vi "GET_LayersLocked_ActiveLayer.vi"(8 "error in (no error)":errorcluster, 11 "Icon.lvclass in":refnum<class "Icon.lvclass">) -> (0 "error out":errorcluster, 1 "Active Layer":i32, 2 "Layers Locked?":bool, 3 "Icon.lvclass out":refnum<class "Icon.lvclass">)   [LabVIEW 2020, in "Icon.lvclass"]
doc: "Returns the active User Layer and whether or not it is locked."
uses:
  Icon.lvclass
  Icon.lvclass/Icon.ctl
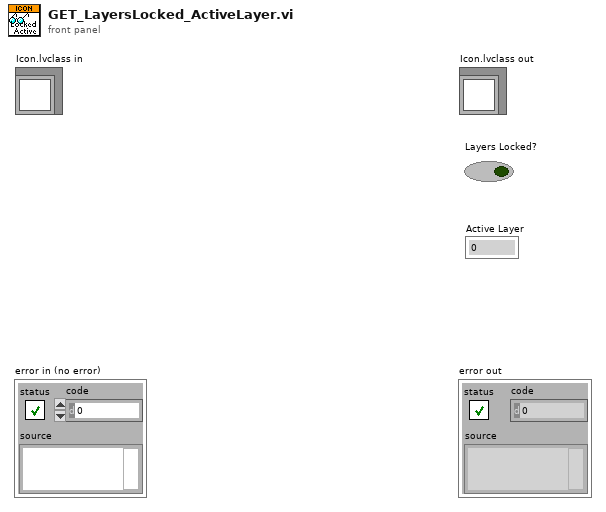
[diagram p1: front panel]
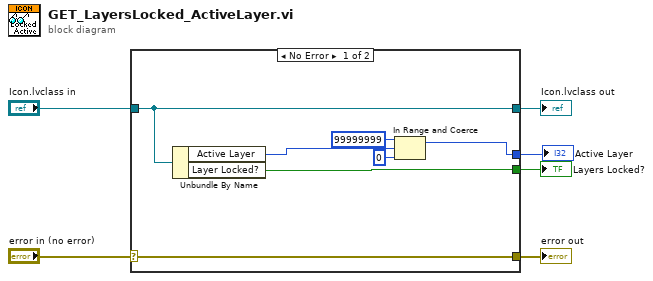
[diagram p0: block diagram]
diagram:
  n1 = case shown="No Error" "error in (no error)" {
    selector: "error in (no error)" -> [w13 w14]
    tunnel: [w13 w14] -> w5
    tunnel: [w12 w15] -> w3
    tunnel: "Icon.lvclass in" -> [w12 w15]
    tunnel: [w11 _] -> w2
    tunnel: [w7 _] -> w1
    frame No Error {
      n2 = Unbundle By Name(w12) -> ("Active Layer"=w10:i32, "Layer Locked?"=w11:bool)
      n3 = In Range and Coerce(upper limit=99999999, x=w10, lower limit=0) -> (coerced(x)=w7:i32)  [unwired: 1 out]
    }
    frame Error {
    }
  }
  "error out" <- w5
  "Icon.lvclass out" <- w3
  "Layers Locked?" <- w2
  "Active Layer" <- w1
